vi "OAT Orbit Plot (Even Angle Signal).vi"(0 "even angle signals":cluster{"r0":dbl, "dr":dbl, "Y":dbl[]}[](array[cluster]) {"r0" format="%.2p"; "dr" format="%.2p"; "Y" format="%.2f"}, 1 "orbit plot ref":refnum<vi>, 2 "reset? (T)":bool=TRUE, 3 "max axis display value":dbl format="%.2f", 5 "speed profile":T1 {"speed [RPM]" format="%.2f"; "time [s]" format="%.2f"}, 7 "even angle position info":T3, 9 "revolutions to display [rev]":cluster{"start":dbl, "duration":dbl}={"start"=0.0, "duration"=1.0} {"duration" format="%.2f"; "start" format="%.2f"}, 11 "error in (no error)":errorcluster, 12 "channel settings":T2={"shaft rotating direction"=0, "probe angles [deg]"={"X"=0, "Y"=90}} {"probe angles [deg]"."Y" max=360 step=1; "probe angles [deg]"."X" max=360 step=1; "shaft rotating direction" items=["CCW", "CW"]}, 14 "trigger pulse direction":u16(ring)=1 items=["positive going", "negative going"]) -> (4 "orbit plot":T4, 15 "error out":errorcluster)   [LabVIEW 2017]
doc: "Draws an orbit plot on an XY graph. You can use this polymorphic VI to draw an orbit plot with unfiltered or filtered data. Unfiltered data comes from the <B>even angle signals</B> input, filtered data from the <B>magnitudes</B> and <B>phases [phase lag]</B> inputs. The data type you wire to the <B>even angle signals</B> input determines the polymorphic instance to use."
uses:
  <vilib>/addons/Sound and Vibration/Order Analysis/Backward Compatibility/SubVIs/oa_Orbit Plot Control.ctl
  <vilib>/addons/Sound and Vibration/Order Analysis/Misc/OAT Position Info.ctl
  <vilib>/addons/Sound and Vibration/Order Analysis/Tach Process/SubVIs/speed profile.ctl
  <vilib>/addons/Sound and Vibration/Order Analysis/Resample Order Tracking/SoundVib_Resampling.lvlib
  <vilib>/addons/Sound and Vibration/Order Analysis/Tach Process/SoundVib_TachProcess.lvlib
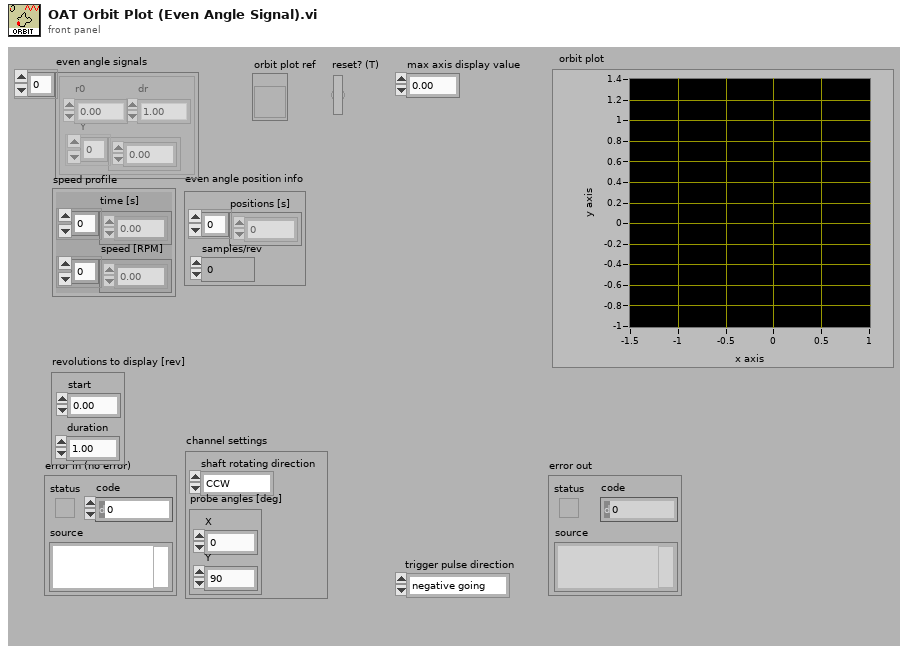
[diagram p1: front panel]
types:
  T1 = typedef "SoundVib_TachProcess.lvlib/speed profile.ctl" = cluster{"time [s]":dbl[], "speed [RPM]":dbl[]}
  T2 = cluster{"shaft rotating direction":u16, "probe angles [deg]":cluster{"X":u32, "Y":u32}}
  T3 = typedef "OAT Position Info.ctl" = cluster{"positions [s]":dbl[], "samples/rev":dbl}
  T4 = typedef "oa_Orbit Plot Control.ctl" = cluster{dbl[], dbl[]}[]
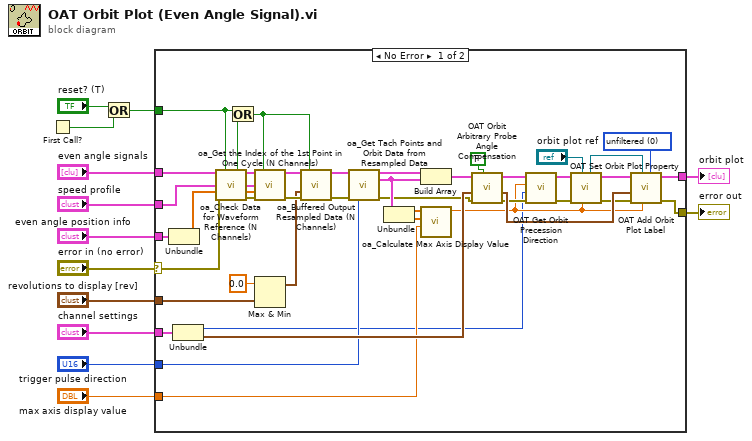
[diagram p0: block diagram]
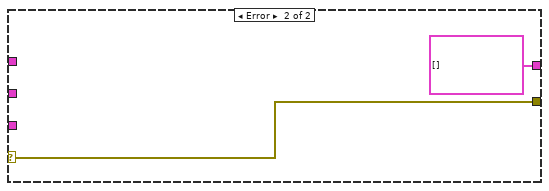
[diagram p2: hidden frame]
diagram:
  n1 = First Call?() -> (First Call?: T/F=w7:bool)
  n2 = Or(x="reset? (T)", y=w7) -> (x .or. y?=w6:bool)
  n3 = case shown="No Error" "error in (no error)" {
    selector: "error in (no error)" -> [w52 w59]
    tunnel: [w18 w59] -> w12
    tunnel: "even angle signals" -> [w53 _]
    tunnel: "speed profile" -> [w51 _]
    tunnel: "even angle position info" -> [w17 _]
    tunnel: w6 -> [w50 _]
    tunnel: "revolutions to display [rev]" -> [w47 _]
    tunnel: [w35 cluster{dbl[], dbl[]}[] [] ("XY plot data out")] -> w4
    tunnel: "channel settings" -> [w34 _]
    tunnel: "trigger pulse direction" -> [w30 _]
    tunnel: "max axis display value" -> [w28 _]
    frame No Error {
      w37 = u16 0 items=["unfiltered", "filtered"] ("plot type")
      n4 = Unbundle(w17) -> ("positions [s]"=w16:dbl[])  [unwired: 1 out]
      n5 = Unbundle(w34) -> ("shaft rotating direction"=w21:u16, "probe angles [deg]"=w33:cluster{"X":u32, "Y":u32})
      n6 = call <vilib>:"oa_Check Data for Waveform Reference (N Channels).vi"("resampled signal"=w53, "reset? (True)"=w50, "speed profile"=w51, "interpolated pulse positions"=w16, "error in (no error)"=w52) -> ("reset"=w49:bool, "resampled data out"=w56:cluster{"r0":dbl, "dr":dbl, "Y":dbl[]}[], "speed profile out"=w54:T1, "interpolated pulse positions out"=w55:dbl[], "error out"=w57:errorcluster)  [unwired: 3 in, 3 out]
      n7 = Or(x=w50, y=w49) -> (x .or. y?=w45:bool)
      n8 = call <vilib>:"oa_Get the Index of the 1st Point in One Cycle (N Channels).vi"("resampled signal"=w56, "reset? (True)"=w45, "speed profile"=w54, "interpolated pulse positions"=w55, "error in (no error)"=w57) -> ("resampled signal out"=w48:cluster{"r0":dbl, "dr":dbl, "Y":dbl[]}[], "error out"=w46:errorcluster)  [unwired: 8 in, 1 out]
      n9 = Max & Min(x=0.0, y=w47) -> (max(x,y)=w14:cluster{"start":dbl, "duration":dbl})  [unwired: 1 out]
      n10 = call <vilib>:"oa_Buffered Output Resampled Data (N Channels).vi"("resampled signal in"=w48, "reset? (True)"=w45, "display revolutions"=w14, "error in"=w46) -> ("resampled signal out"=w32:cluster{"r0":dbl, "dr":dbl, "Y":dbl[]}[], "error out"=w31:errorcluster)  [unwired: 9 in, 1 out]
      n11 = call <vilib>:"oa_Get Tach Points and Orbit Data from Resampled Data.vi"("resampled signal in"=w32, "error in"=w31, "trigger pulse direction"=w30) -> ("tach points"=w29:cluster{dbl[], dbl[]}, "orbit"=w27:cluster{dbl[], dbl[]}, "error out"=w24:errorcluster)  [unwired: 10 in]
      n12 = Unbundle(w27) -> (w26:dbl[], w25:dbl[])
      n13 = Build Array(w29, w27) -> (w40:cluster{dbl[], dbl[]}[])
      n14 = call <vilib>:"oa_Calculate Max Axis Display Value.vi"("max axis display value in"=w28, "orbit data Y"=w25, "orbit data X"=w26) -> ("max data value out"=w22:dbl)  [unwired: 8 in]
      n15 = call <vilib>:"OAT Orbit Arbitrary Probe Angle Compensation.vi"("select methods"=FALSE, "error in (no error)"=w24, "probe angle"=w33, "XY plot data in"=w40) -> ("error out"=w23:errorcluster, "probe angle out"=w39:cluster{"X (red)":dbl, "Y (blue)":dbl}, "XY plot data out"=w44:cluster{dbl[], dbl[]}[])  [unwired: 5 in]
      n16 = call <vilib>:"OAT Get Orbit Precession Direction.vi"("error in (no error)"=w23, "shaft rotating direction"=w21, "max data value"=w22, "XY plot data in"=w44) -> ("error out"=w20:errorcluster, "XY plot data out"=w43:cluster{dbl[], dbl[]}[])  [unwired: 6 in]
      n17 = call <vilib>:"OAT Set Orbit Plot Property.vi"("max value"=w22, "orbit plot ref"="orbit plot ref", "error in (no error)"=w20, "XY plot data in"=w43) -> ("error out"=w19:errorcluster, "XY plot data out"=w42:cluster{dbl[], dbl[]}[], "orbit plot ref"=w41:refnum<vi>)  [unwired: 5 in]
      n18 = call <vilib>:"OAT Add Orbit Plot Label.vi"("plot type"=w37, "max value"=w22, "orbit plot ref"=w41, "error in (no error)"=w19, "probe angle out"=w39, "XY plot data in"=w42) -> ("error out"=w18:errorcluster, "XY plot data out"=w35:cluster{dbl[], dbl[]}[])  [unwired: 4 in]
    }
    frame Error {
    }
  }
  "orbit plot" <- w4
  "error out" <- w12
